vi "IsValid.vi"(11 "String":string) -> (3 "String 2":string)   [LabVIEW 2013, in "main.lvlib"]
uses:
  main.lvlib
  <vilib>/regexp/Match Regular Expression.xnode
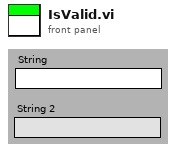
[diagram p1: front panel]
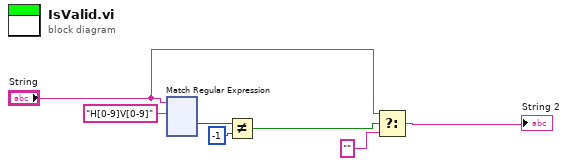
[diagram p0: block diagram]
diagram:
  n1 = xnode "Match Regular Expression"("input string"="String", "regular expression"="H[0-9]V[0-9]") -> ("offset past match"=w6:i32)  [unwired: 4 in, 4 out]
  n2 = Not Equal?(x=w6, y=-1) -> (x != y?=w4:bool)
  n3 = Select(t="String", s=w4, f="") -> (s? t:f=→"String 2":string)
